vi "sub vi - AI USB4704 (3) v71.vi"() -> (1 "Graph 1":waveform(dbl)[](graph), 2 "Graph 2":waveform(dbl)[](graph), 3 "Graph 3":waveform(dbl)[](graph), 10 "loop time":dbl format="%.6g", 15 "error array":errorcluster[](array[cluster]))   [LabVIEW 2013]
uses:
  program files/Global 1.vi
  <userlib>/DAQNavi Polymorphic VI/create/DAQNavi Create Channel(AI-Voltage).vi
  <userlib>/DAQNavi Polymorphic VI/configure/timing/DAQNavi Timing(Convert Clock).vi
  <userlib>/DAQNavi Polymorphic VI/read/DAQNavi Read (Analog 1D Wfm NChan NSamp).vi
panel:
  in  "SAMPLES":dbl
  in  "RATE(Hz)":dbl
  in  "Tab Control":enum32{"USB #0", "USB #1", "USB #2"}(tab)
  out "physical channels 0":string="DemoDevice,BID#0/ai0:1" caption="property value"
  out "value range 0":string="+/- 5 V" caption="property value"
  out "physical channels 1":string="DemoDevice,BID#0/ai0:1" caption="property value"
  out "value range 1":string="+/- 5 V" caption="property value"
  out "physical channels 2":string="DemoDevice,BID#0/ai0:1" caption="property value"
  out "value range 2":string="+/- 5 V" caption="property value"
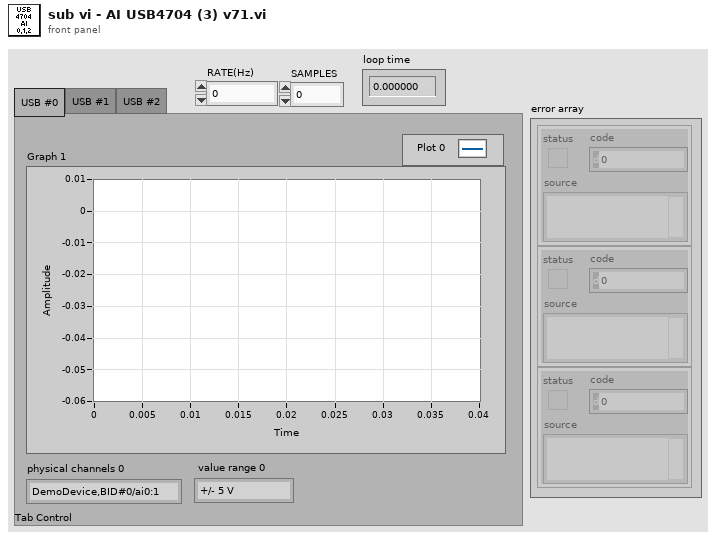
[diagram p1: front panel]
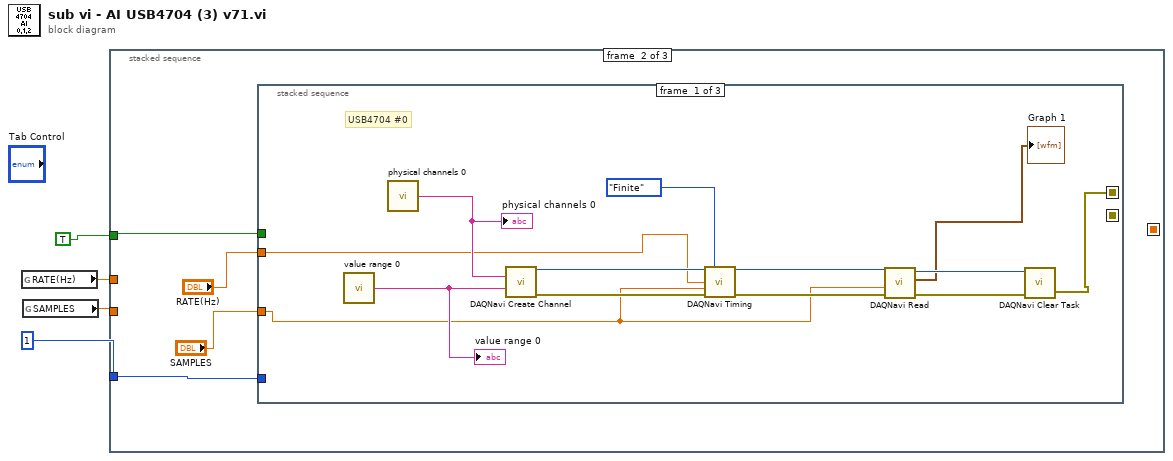
[diagram p0: block diagram]
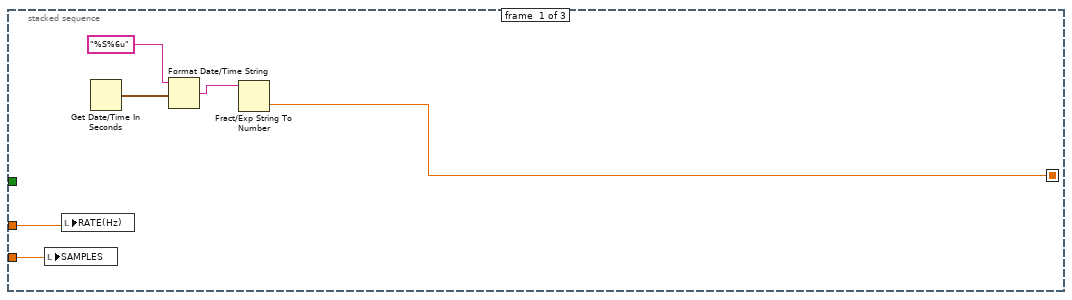
[diagram p2: hidden frame]
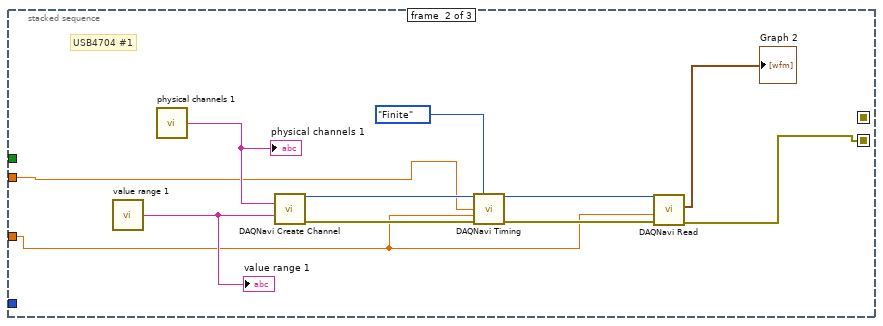
[diagram p3: hidden frame]
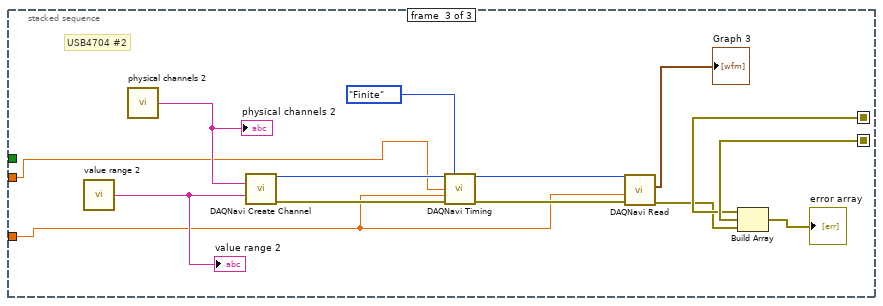
[diagram p4: hidden frame]
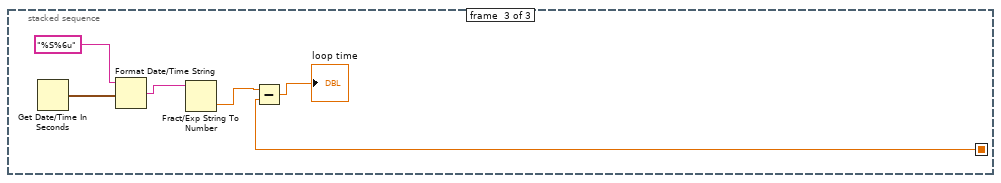
[diagram p5: hidden frame]
diagram:
  n1 = global read "Global 1.vi" "RATE(Hz)"() -> (w3:dbl)
  n2 = global read "Global 1.vi" "SAMPLES"() -> (w2:dbl)
  n3 = stacked-sequence {
    seq-local: [w7 _ _] -> [_ _ w54]
    tunnel: TRUE -> [_ w14 _]
    tunnel: 1 -> [_ w13 _]
    tunnel: w2 -> [w5 _ _]
    tunnel: w3 -> [w6 _ _]
    frame #0 {
      n4 = local write "SAMPLES"(w5) -> ()
      n5 = local write "RATE(Hz)"(w6) -> ()
      n6 = Get Date/Time In Seconds() -> (seconds since 1Jan1904=w9:timestamp)
      n7 = Format Date/Time String(time format string (%c)="%S%6u", seconds (now)=w9) -> (date/time string=w8:string)  [unwired: 1 in]
      n8 = Fract/Exp String To Number(string=w8) -> (number=w7:dbl)  [unwired: 3 in, 1 out]
    }
    frame #1 {
      n9 = stacked-sequence {
        seq-local: [w18 _ _] -> [_ _ w50]
        seq-local: [_ w28 _] -> [_ _ w51]
        tunnel: w14 -> [_ _ _]
        tunnel: "RATE(Hz)" -> [w15 w31 w42]
        tunnel: "SAMPLES" -> [w16 w30 w41]
        tunnel: w13 -> [_ _ _]
        frame #0 {
          # "USB4704 #0"
          n10 = call "value range 0"() -> ("property value"=w19:string)  [unwired: 1 out]
          "value range 0" <- w19
          n11 = call "physical channels 0"() -> ("property value"=w20:string)  [unwired: 1 out]
          "physical channels 0" <- w20
          n12 = call-poly <userlib>:"DAQNavi Create Channel.vi"("physical channels"=w20, "value range"=w19) -> ("task out"=w25:i32, "error out"=w24:errorcluster)  [unwired: 3 in, 9 out]
          n13 = call-poly <userlib>:"DAQNavi Timing.vi"("task in"=w25, "sample mode"=enum16{"Finite", "Continuous"}."Finite", "rate"=w15, "samples per channel"=w16, "error in (no error)"=w24) -> ("task out"=w23:i32, "error out"=w22:errorcluster)  [unwired: 1 in, 8 out]
          n14 = call-poly <userlib>:"DAQNavi Read.vi"("error in (no error)"=w22, "number of samples per channel to read"=w16, "task in"=w23) -> ("error out"=w26:errorcluster, "data"=→"Graph 1":waveform(dbl)[], "task out"=w27:i32)  [unwired: 1 in, 5 out]
          n15 = call <userlib>:"DAQNavi Clear Task.vi"("error in (no error)"=w26, "task in"=w27) -> ("error out"=w18:errorcluster)  [unwired: 1 out]
        }
        frame #1 {
          # "USB4704 #1"
          n16 = call "value range 1"() -> ("property value"=w32:string)  [unwired: 1 out]
          "value range 1" <- w32
          n17 = call "physical channels 1"() -> ("property value"=w33:string)  [unwired: 1 out]
          "physical channels 1" <- w33
          n18 = call-poly <userlib>:"DAQNavi Create Channel.vi"("physical channels"=w33, "value range"=w32) -> ("task out"=w38:i32, "error out"=w37:errorcluster)  [unwired: 3 in, 9 out]
          n19 = call-poly <userlib>:"DAQNavi Timing.vi"("task in"=w38, "sample mode"=enum16{"Finite", "Continuous"}."Finite", "rate"=w31, "samples per channel"=w30, "error in (no error)"=w37) -> ("task out"=w36:i32, "error out"=w35:errorcluster)  [unwired: 1 in, 8 out]
          n20 = call-poly <userlib>:"DAQNavi Read.vi"("error in (no error)"=w35, "number of samples per channel to read"=w30, "task in"=w36) -> ("error out"=w28:errorcluster, "data"=→"Graph 2":waveform(dbl)[])  [unwired: 1 in, 6 out]
        }
        frame #2 {
          # "USB4704 #2"
          n21 = call "value range 2"() -> ("property value"=w43:string)  [unwired: 1 out]
          "value range 2" <- w43
          n22 = call "physical channels 2"() -> ("property value"=w44:string)  [unwired: 1 out]
          "physical channels 2" <- w44
          n23 = call-poly <userlib>:"DAQNavi Create Channel.vi"("physical channels"=w44, "value range"=w43) -> ("task out"=w49:i32, "error out"=w48:errorcluster)  [unwired: 3 in, 9 out]
          n24 = call-poly <userlib>:"DAQNavi Timing.vi"("task in"=w49, "sample mode"=enum16{"Finite", "Continuous"}."Finite", "rate"=w42, "samples per channel"=w41, "error in (no error)"=w48) -> ("task out"=w47:i32, "error out"=w46:errorcluster)  [unwired: 1 in, 8 out]
          n25 = call-poly <userlib>:"DAQNavi Read.vi"("error in (no error)"=w46, "number of samples per channel to read"=w41, "task in"=w47) -> ("error out"=w40:errorcluster, "data"=→"Graph 3":waveform(dbl)[])  [unwired: 1 in, 6 out]
          n26 = Build Array(w50, w51, w40) -> (→"error array":errorcluster[])
        }
      }
    }
    frame #2 {
      n27 = Get Date/Time In Seconds() -> (seconds since 1Jan1904=w57:timestamp)
      n28 = Format Date/Time String(time format string (%c)="%S%6u", seconds (now)=w57) -> (date/time string=w56:string)  [unwired: 1 in]
      n29 = Fract/Exp String To Number(string=w56) -> (number=w55:dbl)  [unwired: 3 in, 1 out]
      n30 = Subtract(x=w55, y=w54) -> (x-y=→"loop time":dbl)
    }
  }
